vi "Verify new image.vi"(8 "error in (no error)":errorcluster, 11 "CCDCamera in":refnum<class "Simulated_CCD_Camera.lvclass">) -> (0 "error out":errorcluster, 2 "New Images ?":bool, 3 "CCDCamera out":refnum<class "Simulated_CCD_Camera.lvclass">)   [LabVIEW 2018, in "Simulated_CCD_Camera.lvclass"]
doc: "Verify is there is any new image"
uses:
  Simulated_CCD_Camera.lvclass
  Simulated_CCD_Camera.lvclass/Simulated_CCD_Camera.ctl
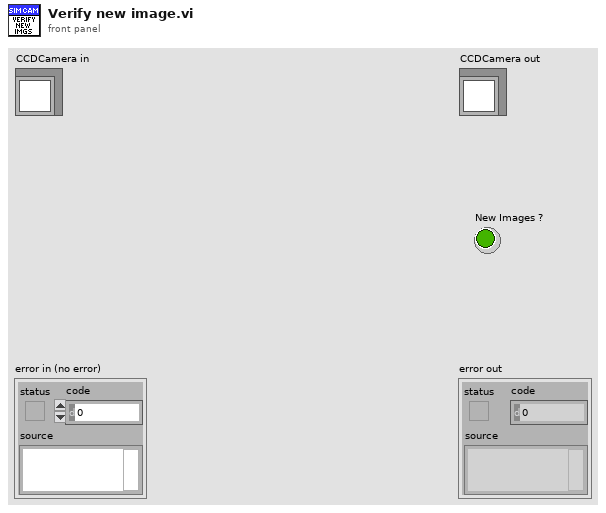
[diagram p1: front panel]
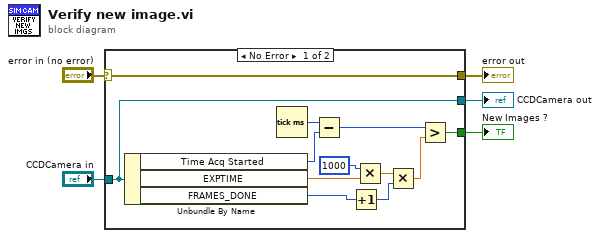
[diagram p0: block diagram]
diagram:
  n1 = case shown="No Error" "error in (no error)" {
    selector: "error in (no error)" -> [w8 w19]
    tunnel: [w8 w19] -> w4
    tunnel: [w17 w18] -> w2
    tunnel: "CCDCamera in" -> [w17 w18]
    tunnel: [w9 _] -> w1
    frame No Error {
      n2 = Unbundle By Name(w17) -> ("Time Acq Started"=w14:u32, "EXPTIME"=w7:dbl, "FRAMES_DONE"=w6:u16)
      n3 = Tick Count (ms)() -> (millisecond timer value=w15:u32)
      n4 = Subtract(x=w15, y=w14) -> (x-y=w11:u32)
      n5 = Increment(x=w6) -> (x+1=w12:u16)
      n6 = Multiply(x=1000, y=w7) -> (x*y=w13:dbl)
      n7 = Multiply(x=w13, y=w12) -> (x*y=w10:dbl)
      n8 = Greater?(x=w11, y=w10) -> (0:w9:bool)
    }
    frame Error {
    }
  }
  "error out" <- w4
  "CCDCamera out" <- w2
  "New Images ?" <- w1
